vi "Num Ref Get DBL String.vi"(8 "error in (no error)":errorcluster, 11 "DBL Ref":refnum<vi>) -> (0 "error out":errorcluster, 3 "Value string":string)   [LabVIEW 2018, in "Main Panel.lvlib" / "Main Panel.lvclass"]
uses:
  Main Panel.lvclass
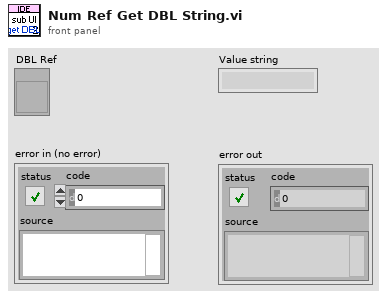
[diagram p1: front panel]
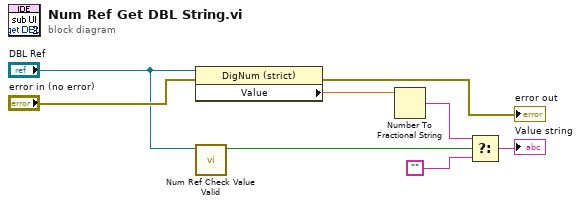
[diagram p0: block diagram]
diagram:
  n1 = property class="DigNum (strict)"(reference="DBL Ref", error in="error in (no error)") -> (error out=→"error out":errorcluster, "Value"=w2:dbl)  [unwired: 1 out]
  n2 = call "Num Ref Check Value Valid.vi"("Num Ref"="DBL Ref") -> ("Valid"=w7:bool)  [unwired: 9 in, 1 out]
  n3 = Number To Fractional String(number=w2) -> (F-format string=w1:string)  [unwired: 3 in]
  n4 = Select(t=w1, s=w7, f="") -> (s? t:f=→"Value string":string)
